vi "Render Section Children.vi"(8 "Error In":errorcluster, 10 "Section":refnum<class "Section.lvclass">, 11 "Context In":refnum<class "Context.lvclass">) -> (0 "Error Out":errorcluster, 2 "Output":string, 3 "Context Out":refnum<class "Context.lvclass">)   [LabVIEW 2018, in "Toolkit.lvlib"]
uses:
  Toolkit.lvlib
  Context/Context.lvclass
  Nodes/Section/Section.lvclass
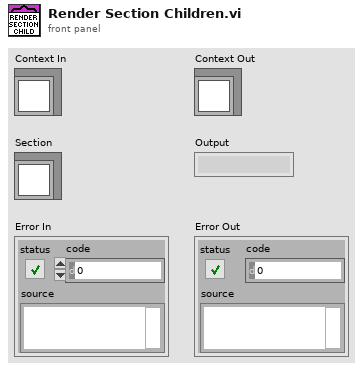
[diagram p1: front panel]
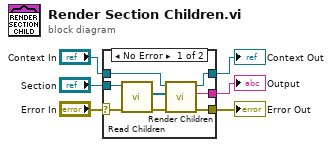
[diagram p0: block diagram]
diagram:
  n1 = case shown="No Error" "Error In" {
    selector: "Error In" -> [w13 w16]
    tunnel: [w9 w16] -> w6
    tunnel: "Context In" -> [w11 w15]
    tunnel: "Section" -> [w14 _]
    tunnel: [w10 w15] -> w2
    tunnel: [w7 _] -> w1
    frame No Error {
      n2 = call-dynamic "Read Children.vi"("Error In"=w13, "NonTerminal In"=w14) -> ("Error Out"=w8:errorcluster, "Children"=w12:refnum<class "Abstract.lvclass">[])  [unwired: 7 in, 1 out]
      n3 = call "Render Children.vi"("Error In"=w8, "Children"=w12, "Context In"=w11) -> ("Error Out"=w9:errorcluster, "Output"=w7:string, "Context Out"=w10:refnum<class "Context.lvclass">)  [unwired: 6 in]
    }
    frame Error {
    }
  }
  "Output" <- w1
  "Error Out" <- w6
  "Context Out" <- w2
